vi "HRM-process-filter_waveform.vi"(8 "error in (no error)":errorcluster, 11 "Process data":T1={"Raw collected data"={"t0"=timestamp(0 s since 1904-01-01), "dt"=1.0, "Y"=[]}, "filtered data"={"t0"=timestamp(0 s since 1904-01-01), "dt"=1.0, "Y"=[]}, "Heartrate"=0.0, "Additional Signal to remove [s]"=0, "samples [s]"=10, "Pulse settings"={"Manual?"=FALSE, "Top"=0.0, "Bottom"=0.0}, "User Events"={"Additional Signal to remove [s]"=refnum, "samples [s]"=refnum, "Heart Rate"=refnum, "Raw collected data"=refnum, "Filtered data"=refnum, "Raw Data"=refnum, "stop"=refnum, "Status Feedback"=refnum, "pause AQN"=refnum, "Clear wf Data"=refnum, "Pulse settings"=refnum}}) -> (0 "error out":errorcluster, 3 "Process data ouy":T1={"Raw collected data"={"t0"=timestamp(0 s since 1904-01-01), "dt"=1.0, "Y"=[]}, "filtered data"={"t0"=timestamp(0 s since 1904-01-01), "dt"=1.0, "Y"=[]}, "Heartrate"=0.0, "Additional Signal to remove [s]"=0, "samples [s]"=10, "Pulse settings"={"Manual?"=FALSE, "Top"=0.0, "Bottom"=0.0}, "User Events"={"Additional Signal to remove [s]"=refnum, "samples [s]"=refnum, "Heart Rate"=refnum, "Raw collected data"=refnum, "Filtered data"=refnum, "Raw Data"=refnum, "stop"=refnum, "Status Feedback"=refnum, "pause AQN"=refnum, "Clear wf Data"=refnum, "Pulse settings"=refnum}})   [LabVIEW 2020]
uses:
  HRM-process-loop_data.ctl
  HRM-process-Pulse settings.ctl
  init/HRM-init-user_events.ctl
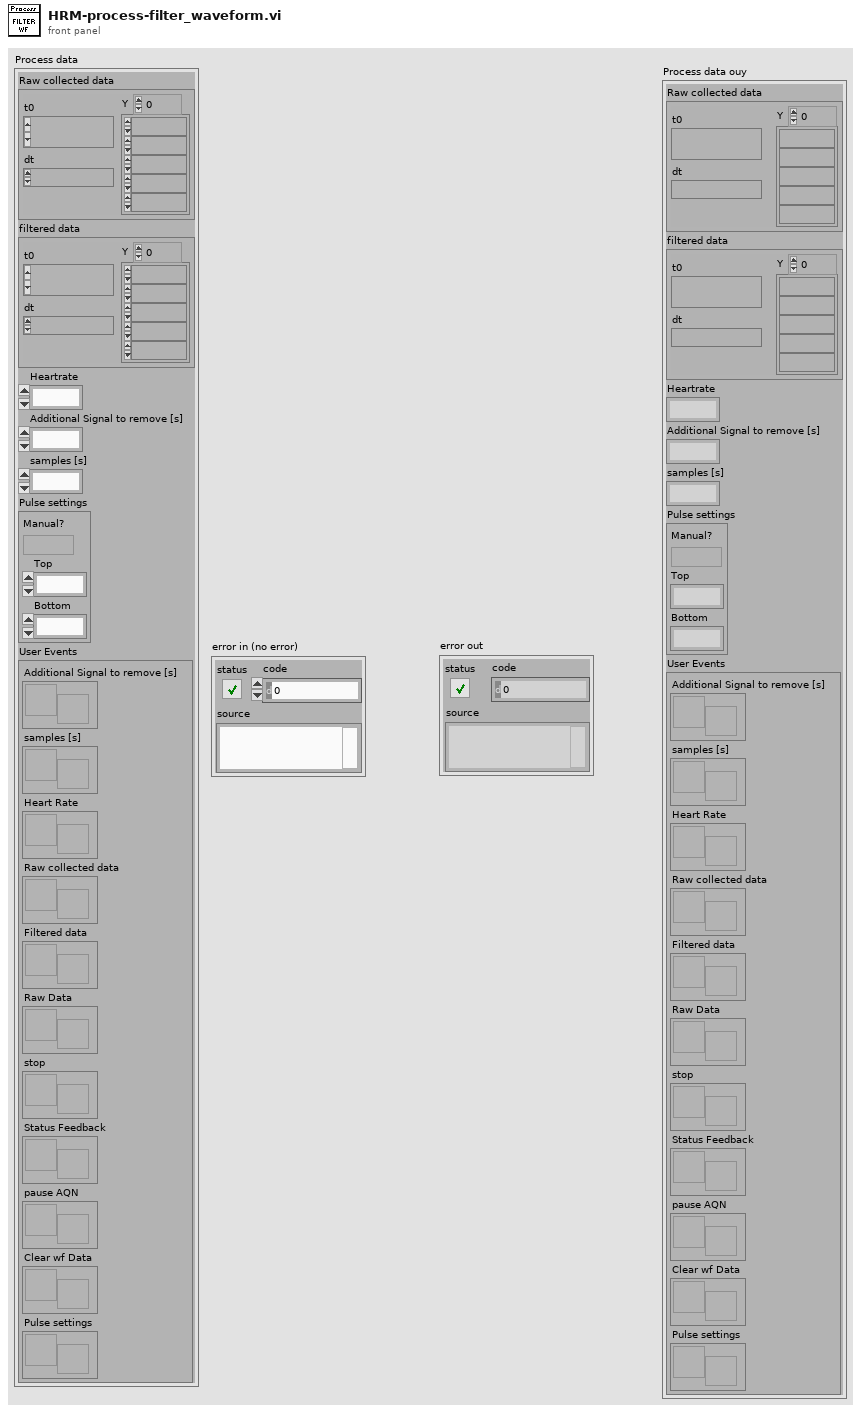
[diagram p1: front panel]
types:
  T1 = typedef "HRM-process-loop_data.ctl" = cluster{"Raw collected data":waveform(dbl), "filtered data":waveform(dbl), "Heartrate":dbl, "Additional Signal to remove [s]":i32, "samples [s]":i32, "Pulse settings":T2, "User Events":T3}
  T2 = typedef "HRM-process-Pulse settings.ctl" = cluster{"Manual?":bool, "Top":dbl, "Bottom":dbl}
  T3 = typedef "HRM-init-user_events.ctl" = cluster{"Additional Signal to remove [s]":refnum<user-event>, "samples [s]":refnum<user-event>, "Heart Rate":refnum<user-event>, "Raw collected data":refnum<user-event>, "Filtered data":refnum<user-event>, "Raw Data":refnum<user-event>, "stop":refnum<user-event>, "Status Feedback":refnum<user-event>, "pause AQN":refnum<user-event>, "Clear wf Data":refnum<user-event>, "Pulse settings":refnum<user-event>}
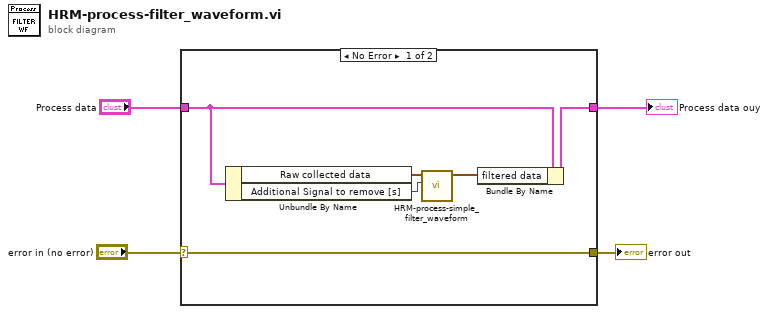
[diagram p0: block diagram]
diagram:
  n1 = case shown="No Error" "error in (no error)" {
    selector: "error in (no error)" -> [w10 w11]
    tunnel: [w10 w11] -> w3
    tunnel: "Process data" -> [w8 w12]
    tunnel: [w9 w12] -> w1
    frame No Error {
      n2 = Unbundle By Name(w8) -> ("Raw collected data"=w7:waveform(dbl), "Additional Signal to remove [s]"=w5:i32)
      n3 = call "HRM-process-simple_filter_waveform.vi"("Additional Signal to remove [s]"=w5, "data in"=w7) -> ("data out"=w6:waveform(dbl))  [unwired: 9 in]
      n4 = Bundle By Name(cluster=w8, "filtered data"=w6) -> (w9:T1)
    }
    frame Error {
    }
  }
  "Process data ouy" <- w1
  "error out" <- w3
